vi "Spike-LEGO.vi"() -> ()   [LabVIEW 2016]
uses:
  VIs/uPythonX/uPythonX.xctl
panel:
  in  "Tab Control":T1(tab)
  in  "uPythonX":T2(xcontrol)={"VISA Refnum in"="ASRL75::INSTR", "Python Code"="import hub\n\nhub.firmware.bootloader_version()\n# 'v0.5.01.0000-42a938e'\n\nhub.firmware.info()\n\nhub.info()"}
  in  "Battery":T3(xcontrol)={"VISA Refnum in"="ASRL48::INSTR", "All Code"="'''\nThe Hub battery is chargable and readout of various values related to the battery is provided.\n'''\n\nfrom hub import battery\n\n# get all info - returns error state, charger state, voltage, filtered voltage, temperature, current and capacity left\n\nbattery.info()\n\n\n'''\nerror_state - \n     battery.BATTERY_NO_ERROR = 0\n     battery.BATTERY_HUB_TEMPERATURE_CRITICAL_OUT_OF_RANGE = -1\n     battery.BATTERY_TEMPERATURE_OUT_OF_RANGE = -2\n     battery.BATTERY_TEMPERATURE_SENSOR_FAIL = -3\n     battery.BATTERY_BAD_BATTERY = -4\n     battery.BATTERY_VOLTAGE_TOO_LOW = -5\n\ncharger_state - The state of the charter circuit:\n     battery.DISCHARGING = 0\n     battery.CHARGING_ONGOING = 1\n     battery.CHARGING_COMPLETED = 2\n     battery.FAIL = -1\n\ncharge_voltage - The battery volgate in mV\n\ncharge_voltage_filtered - The battery volgate (filtered) in mV\n\ntemperature - The battery temperature in degree Celcius.\n\ncharge_current - The battery charging current in mA (the current flowing into the battery)\n\nbattery_capacity_left - The battery capacity left in percent of full capacity\n\n'''\n\n\n"}
  in  "Buttons":T3(xcontrol)={"VISA Refnum in"="ASRL48::INSTR", "All Code"="'''\nThe buttons on the front of the Hub are used to navigate the UI in \nSelection mode, and can be used to interact with the user in the Run mode. \nThere are 4 buttons left, center, right, connect\n'''\n\nimport hub\n\n# can ask if it is currently pressed, was pressed, how many times it has been pressed, and callback\n\nwhile True:\n    if hub.button.left.is_pressed():\n        hub.display.show(hub.Image.YES)\n    elif hub.button.right.is_pressed():\n        hub.display.show(hub.Image.NO)\n        \n# possible buttons are left, center, right, connect\n\nhub.button.center.is_pressed()  # checks current state of center button\n\nhub.button.center.was_pressed()  # checks if the  center button has been pressed since last checked\n\nhub.button.center.presses()  # returns # presses since last call and rezeros\n\ndef smile():\n     hub.display.show(hub.Image.SMILE)\n     \nsmile()\n\n#This is not working for me for some reason\nhub.button.center.on_change(smile())  # smiles when button pressed\n\n"}
  in  "Display":T3(xcontrol)={"VISA Refnum in"="ASRL41::INSTR", "All Code"="'''\nThis module controls the 5×5 LED display on the front of the hub. \nIt can be used to display images, animations and even text.\n'''\n\nimport hub,utime\n\n# can display scrolling text or stationary images\n\nhub.display.show(hub.Image.HAPPY)\n\n# You can wait until the previous things is done with  clear=True\n\n# sample callback\n\ndef beep():\n     hub.sound.volume(10)\n     hub.sound.beep(2000, 500, 3)\n\nhub.display.show('LEGO ', loop=False, delay=500, clear = True, fade = 0, callback = beep())\n\n# you can set individual ixels\n\nhub.display.set_pixel(2,3,9)  # x,y, brightness - 0-9\n\nhub.display.get_pixel(2,3)\n\nhub.display.clear()\n\nhub.display.rotation(90)    # can be 0, 90, 180, 270\nhub.display.show(hub.Image.HAPPY)\nutime.sleep_ms(3000)\nhub.display.rotation(0)\nhub.display.show(hub.Image.HAPPY)\n\n\nhub.display.show([hub.Image(\"09090:99999:99999:09990:00900\"),hub.Image(\"01010:11111:11111:01110:00100\")],fade=2,loop=1,delay=500)\n\nhub.display.show(hub.Image.ALL_CLOCKS, loop=True, delay=100)  # note loops forever\n\nhub.display.show('LEGO ', loop=True, delay=500)\n\nhub.display.show('LEGO ', loop=True, fade=4, delay=1000)\n\nhub.display.show(hub.Image.HAPPY, fade=5, delay=2000)\n\nhub.display.show(hub.Image.HAPPY, fade=6, delay=2000)"}
  in  "Image":T3(xcontrol)={"VISA Refnum in"="ASRL41::INSTR", "All Code"="'''\nThe Image clas is used to create images that can be displayed easily on the \n     device’s LED matrix.\n'''\nimport hub, utime\nhub.display.show(hub.Image.HAPPY)\n\nimage = hub.Image(\"90009:\"\n                      \"09090:\"\n                      \"00900:\"\n                      \"09090:\"\n                      \"90009\")    \n\nhub.display.show(image)\nutime.sleep(1)\n\n# or\n\nimage = hub.Image(\"90009\\n09090\\n00900\\n09090\\n90009\")\n\nhub.display.show(image)\nutime.sleep(1)\n\nimage = hub.Image(2, 2, b'\\x08\\x08\\x08\\x08')\n\nhub.display.show(image)\nutime.sleep(1)\n\n# all not working\nhub.Image.width()\nhub.Image.height()\nhub.Image.get_pixel(2,3)\n\nhub.Image.set_pixel(3,1,6)  # you cannot do this on built-in images\n\n'''\nbuilt-in images\n\nImage.HEART\nImage.HEART_SMALL\nImage.HAPPY\nImage.SMILE\nImage.SAD\nImage.CONFUSED\nImage.ANGRY\nImage.ASLEEP\nImage.SURPRISED\nImage.SILLY\nImage.FABULOUS\nImage.MEH\nImage.YES\nImage.NO\nImage.CLOCK12, Image.CLOCK11, Image.CLOCK10, Image.CLOCK9, Image.CLOCK8, Image.CLOCK7, Image.CLOCK6, Image.CLOCK5, Image.CLOCK4, Image.CLOCK3, Image.CLOCK2, Image.CLOCK1\nImage.ARROW_N, Image.ARROW_NE, Image.ARROW_E, Image.ARROW_SE, Image.ARROW_S, Image.ARROW_SW, Image.ARROW_W, Image.ARROW_NW\nImage.TRIANGLE\nImage.TRIANGLE_LEFT\nImage.CHESSBOARD\nImage.DIAMOND\nImage.DIAMOND_SMALL\nImage.SQUARE\nImage.SQUARE_SMALL\nImage.RABBIT\nImage.COW\nImage.MUSIC_CROTCHET\nImage.MUSIC_QUAVER\nImage.MUSIC_QUAVERS\nImage.PITCHFORK\nImage.XMAS\nImage.PACMAN\nImage.TARGET\nImage.TSHIRT\nImage.ROLLERSKATE\nImage.DUCK\nImage.HOUSE\nImage.TORTOISE\nImage.BUTTERFLY\nImage.STICKFIGURE\nImage.GHOST\nImage.SWORD\nImage.GIRAFFE\nImage.SKULL\nImage.UMBRELLA\nImage.SNAKE\n\nFinally, related collections of images have been grouped together:\n\nImage.ALL_CLOCKS\nImage.ALL_ARROWS\n'''"}
  in  "LED":T3(xcontrol)={"VISA Refnum in"="ASRL48::INSTR", "All Code"="'''\nThe user RGB LED capabilities of the hub is a pair of RGB LEDs on \n      either side of the center button.\n'''\nimport hub,utime\n\nhub.led(255, 0, 0) # red  (r,g,b)\n\nhub.led(3) # blue   (colors 0 - 10)\n\nhub.led\n\nfor i in range(11):\n     hub.led(i)\n     utime.sleep(1)\n"}
  in  "Motion":T3(xcontrol)={"VISA Refnum in"="ASRL48::INSTR", "All Code"="'''\nMotion is an object that controls the movement sensors.\n'''\n\nimport hub,utime\n\nhub.motion.accelerometer()\n\nhub.motion.gyroscope()\n\nhub.motion.position()\n\nhub.motion.orientation()  # has a callback option\n\ndef beep():\n     hub.sound.volume(10)\n     hub.sound.beep(2000, 500, 3)\n\nhub.motion.callback(beep())\n\nhub.motion.gesture('down')  # is it currently active?\n\nhub.motion.was_gesture('down')  # has it been active since the last call?\n\n\n\n'''\npossible gestures:\n\nleftside\nrightside\ndown\nup\nfront\nback\ntapped\ndoubletapped\nshake\nfreefall\n'''"}
  in  "Motor":T3(xcontrol)={"VISA Refnum in"="ASRL48::INSTR", "All Code"="'''\nThe ports on the hub are able to autodetect the capabilities of \n     the device that is plugged in. \\When a motor device is detected, \n     then an enhanced set of methods is available.\n'''\n\nimport hub,utime\n\nhub.port.A.motor.mode(1)\nhub.port.A.motor.get()\nhub.port.A.motor.pwm(100) # from -100 to 100\nutime.sleep(1)\nhub.port.A.motor.float()\nhub.port.A.motor.brake()\nhub.port.A.motor.run_at_speed(speed = 50, max_power = 100, acceleration = 100, deceleration = 100, stall = False)\nhub.port.A.motor.run_for_degrees(degrees = 90, speed = 50)\nhub.port.A.motor.run_to_position(90, 50)  # position and speed\nhub.port.A.motor.default()\nhub.port.A.motor.run_for_time(100, 50)   # time - msec and speed\n\n\nhub.port.B.info()\n\n# only works if motors are connected\np = hub.port.A.motor.pair(hub.port.B.motor)\np.pwm(40,-40)   # drive straight\np.run_for_time(200,40,-40)\np.float()   # not working yet\n"}
  in  "Sound":T3(xcontrol)={"VISA Refnum in"="ASRL48::INSTR", "All Code"="'''\nThe sound capabilities of the hub are currently limited to generating \n     simple waveforms:\n\nsin\nsquare\ntriangle\nsawtooth\n\nThe volume of the speaker in the low frequency range (800 Hz) is limited\n'''\n\nimport hub,utime\n\nhub.sound.volume()\nhub.sound.volume(10)  # 0 - 10 \nhub.sound.beep()\nhub.sound.beep(2000, 500, 3)  # freq, time, waveform (sin,square,triangle, sawtooth\n\n# can also play files and have a callback when the sound is complete or interrupted\n"}
  in  "main":T3(xcontrol)={"VISA Refnum in"="ASRL41::INSTR", "All Code"="'''\nstarts at 50, \n     left arrow speeds up, \n     right arrow slows down, \n     center button turns on and off and \n     connect ends code\n'''\nimport hub, utime\n\ndef beep():\n     hub.sound.volume(10)\n     hub.sound.beep(500, 500, 3)\n\ndef go(speed):\n     motorPair.pwm(speed,-speed)\n     show(str(speed//10))\n\ndef show(string):\n     hub.display.show(string)\n\n\nmotorPair = hub.port.A.motor.pair(hub.port.B.motor)\ncenterButton = hub.button.center\nconnectButton = hub.button.connect\nleftButton = hub.button.left\nrightButton = hub.button.right\n\nmotors = False\nspeed = 50\n\nbeep()\nwhile not connectButton.was_pressed():\n     if leftButton.was_pressed():\n          speed = speed + 10\n          if speed > 100:\n               speed = 100\n          go(speed)\n     if rightButton.was_pressed():\n          speed = speed - 10\n          if speed < -100:\n               speed = -100\n          go(speed)\n     if centerButton.was_pressed():\n          if motors:\n               motors = False\n               go(0)\n          else:\n               motors = True\n               go(speed)\n     else:\n          utime.sleep(0.5)"}
  in  "main":T3(xcontrol)={"VISA Refnum in"="ASRL41::INSTR", "All Code"="'''\nstarts at 50, \n     left arrow speeds up, \n     right arrow slows down, \n     center button turns on and off and \n     connect ends code\n'''\nimport flipper, utime\n\ndef beep():\n     flipper.sound.volume(10)\n     flipper.sound.beep(500, 500, 3)\n\ndef go(speed):\n     flipper.port_A.pwm(speed)\n     flipper.port_B.pwm(-speed)\n     show(str(speed//10))\n\ndef show(string):\n     flipper.display.show(string)\n\ncenterButton = flipper.button_center\nconnectButton = flipper.button_connect\nleftButton = flipper.button_left\nrightButton = flipper.button_right\n\nmotors = False\nspeed = 50\n\nbeep()\nwhile not connectButton.was_pressed():\n     if leftButton.was_pressed():\n          speed = speed + 10\n          if speed > 100:\n               speed = 100\n          go(speed)\n     if rightButton.was_pressed():\n          speed = speed - 10\n          if speed < -100:\n               speed = -100\n          go(speed)\n     if centerButton.was_pressed():\n          if motors:\n               motors = False\n               go(0)\n          else:\n               motors = True\n               go(speed)\n     else:\n          utime.sleep(0.5)"}
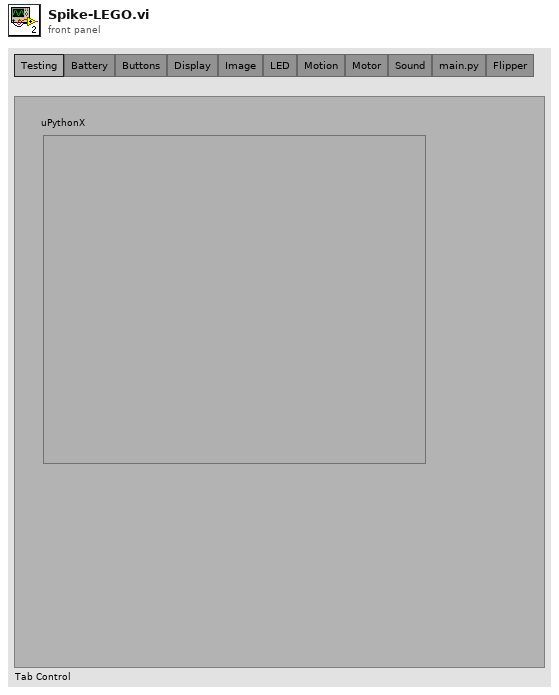
[diagram p1: front panel]
types:
  T1 = enum32{"Testing", "Battery", "Buttons", "Display", "Image", "LED", "Motion", "Motor", "Sound", "main.py", "Flipper"}
  T2 = cluster{"VISA Refnum in":refnum<visa-resource-name>, "Python Code":string}
  T3 = cluster{"VISA Refnum in":refnum<visa-resource-name>, "All Code":string}
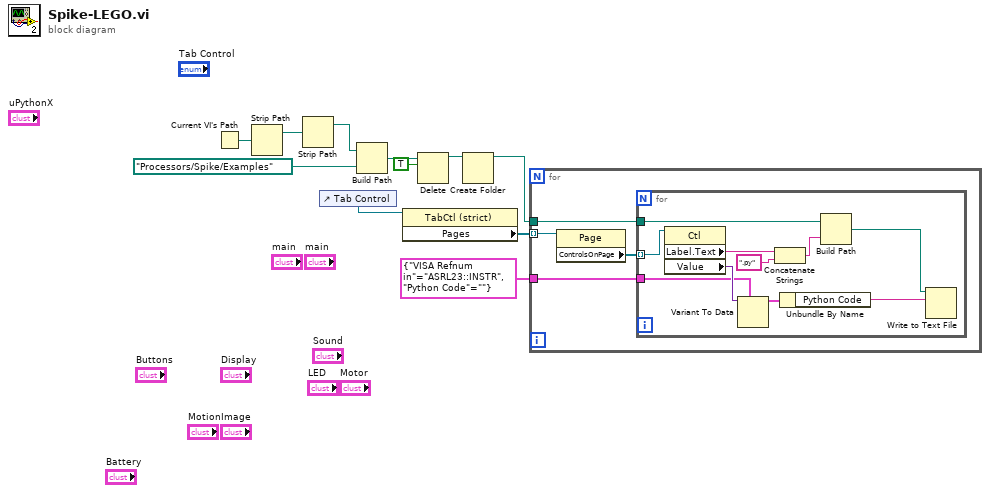
[diagram p0: block diagram]
diagram:
  n1 = Current VI's Path() -> (path=w9:path)
  n2 = Strip Path(path=w9) -> (stripped path=w8:path)  [unwired: 1 out]
  n3 = Strip Path(path=w8) -> (stripped path=w7:path)  [unwired: 1 out]
  n4 = control-ref of="Tab Control"() -> (w1:refnum<vi>)
  n5 = Build Path(base path=w7, name or relative path=path "Processors/Spike/Examples") -> (appended path=w4:path)
  n6 = property class="TabCtl (strict)"(reference=w1) -> ("Pages"=w11:refnum<vi>[])  [unwired: 1 in, 2 out]
  n7 = Delete(path (use dialog)=w4, entire hierarchy (F)=TRUE) -> (deleted path=w3:path)  [unwired: 3 in, 2 out]
  n8 = Create Folder(path (use dialog)=w3) -> (created path=w2:path)  [unwired: 2 in, 2 out]
  n9 = for {
    tunnel: w11 -> [w15] mode=indexing
    tunnel: T2 {"VISA Refnum in"="ASRL23::INSTR", "Python Code"=""} ("VOC") -> [w13]
    tunnel: w2 -> [w12]
    n10 = property class="Page"(reference=w15) -> ("ControlsOnPage"=w14:refnum<vi>[])  [unwired: 1 in, 2 out]
    n11 = for {
      tunnel: w14 -> [w25] mode=indexing
      tunnel: w13 -> [w23]
      tunnel: w12 -> [w21]
      n12 = property class="Ctl"(reference=w25) -> ("Label.Text"=w20:string, "Value"=w24:variant)  [unwired: 1 in, 2 out]
      n13 = Variant To Data(type=w23, Variant=w24) -> (data=w22:T2)  [unwired: 1 in, 1 out]
      n14 = Concatenate Strings(w20, ".py" ("string")) -> (w19:string)
      n15 = Unbundle By Name(w22) -> ("Python Code"=w16:string)
      n16 = Build Path(base path=w21, name or relative path=w19) -> (appended path=w17:path)
      n17 = Write to Text File(file (use dialog)=w17, text=w16) -> ()  [unwired: 2 in, 3 out]
    }
  }
